vi "DB_LeeTHD_Graficas.vi"(8 "error in (no error)":errorcluster, 11 "ID_EQUIPO":i32=1) -> (0 "error out":errorcluster, 3 "THD out":T1)   [LabVIEW 2018]
uses:
  Controls/THD_cluster.ctl
  <vilib>/addons/database/Connection.llb/DB Tools Open Connec (Path).vi
  <vilib>/addons/database/Connection.llb/Conn Execute.vi
  <vilib>/addons/database/Recordset.llb/Rec Fetch Recordset Data (R).vi
  <vilib>/addons/database/Recordset.llb/Rec Destroy - Connection.vi
  <vilib>/addons/database/_DB Variant To Data/Database Variant To Data.xnode
  <vilib>/addons/database/NI_Database_API.lvlib
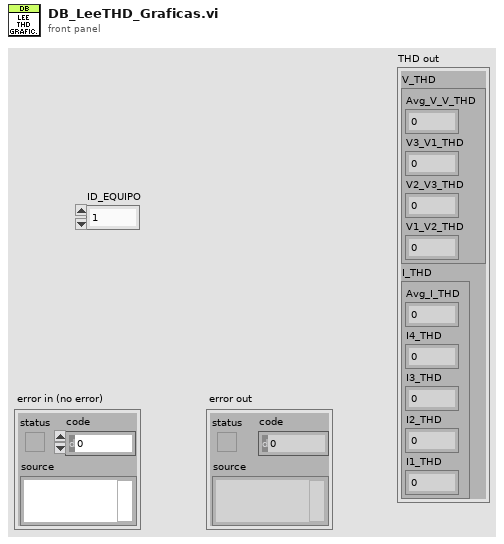
[diagram p1: front panel]
types:
  T1 = typedef "THD_cluster.ctl" = cluster{"V_THD":cluster{"Avg_V_V_THD":sgl, "V3_V1_THD":sgl, "V2_V3_THD":sgl, "V1_V2_THD":sgl}, "I_THD":cluster{"Avg_I_THD":sgl, "I4_THD":sgl, "I3_THD":sgl, "I2_THD":sgl, "I1_THD":sgl}}
  T2 = cluster{"Avg_I_THD":sgl, "I4_THD":sgl, "I3_THD":sgl, "I2_THD":sgl, "I1_THD":sgl}
  T3 = cluster{"Avg_V_V_THD":sgl, "V3_V1_THD":sgl, "V2_V3_THD":sgl, "V1_V2_THD":sgl}
  T4 = typedef "NI_Database_API.lvlib/Conn ObjectReference.ctl" = refnum<k1>
  T5 = typedef "NI_Database_API.lvlib/Rec ObjectReference.ctl" = refnum<k1>
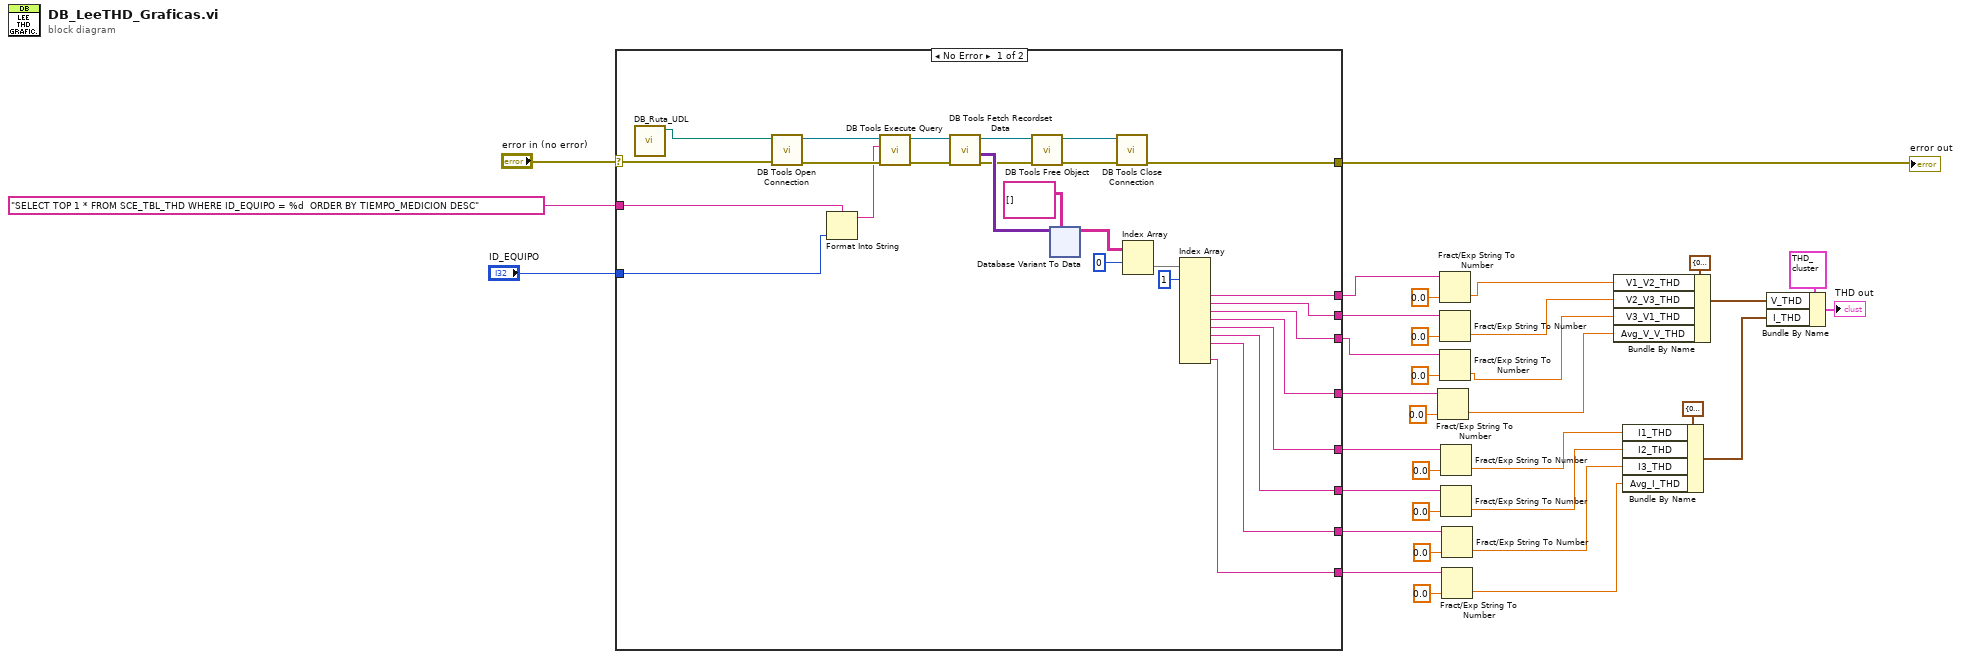
[diagram p0: block diagram]
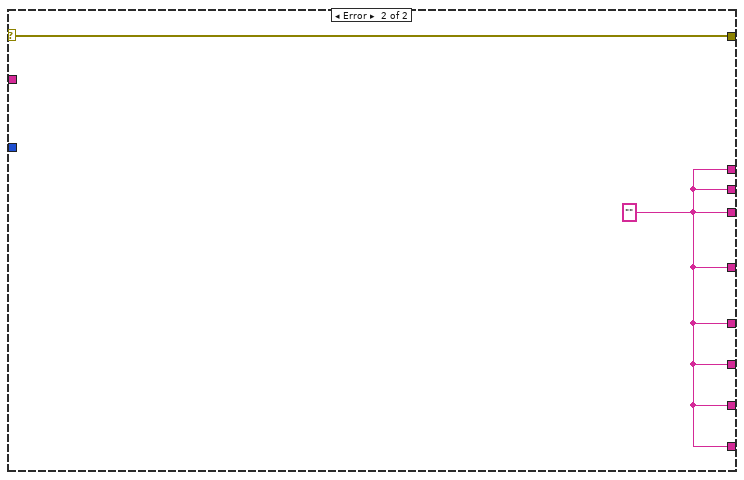
[diagram p2: hidden frame]
diagram:
  n1 = case shown="No Error" "error in (no error)" {
    selector: "error in (no error)" -> [w57 w108]
    tunnel: [w59 w108] -> w32
    tunnel: "SELECT TOP 1 * FROM SCE_TBL_THD WHERE ID_EQUIPO = %d  ORDER BY TIEMPO_MEDICION DESC" ("SQL") -> [w49 _]
    tunnel: [w45 w107] -> w30
    tunnel: [w44 w107] -> w26
    tunnel: [w43 w107] -> w25
    tunnel: "ID_EQUIPO" -> [w46 _]
    tunnel: [w41 w107] -> w21
    tunnel: [w42 w107] -> w20
    tunnel: [w40 w107] -> w19
    tunnel: [w38 w107] -> w9
    tunnel: [w37 w107] -> w7
    frame No Error {
      n2 = call "DB_Ruta_UDL.vi"() -> ("UDL ruta"=w36:path)  [unwired: 11 in]
      n3 = call-poly <vilib>:"DB Tools Open Connection.vi"("error in (no error)"=w57, "connection information"=w36) -> ("error out"=w62:errorcluster, "connection reference"=w60:T4)  [unwired: 6 in]
      n4 = Format Into String(format string=w49, w46) -> (resulting string=w48:string)  [unwired: 2 in, 1 out]
      n5 = call-poly <vilib>:"DB Tools Execute Query.vi"("error in (no error)"=w62, "SQL query"=w48, "connection reference"=w60) -> ("error out"=w58:errorcluster, "recordset reference"=w56:T5)  [unwired: 5 in]
      n6 = call-poly <vilib>:"DB Tools Fetch Recordset Data.vi"("error in (no error)"=w58, "recordset reference"=w56) -> ("error out"=w52:errorcluster, "recordset data"=w53:variant[][], "recordset reference out"=w55:T5)  [unwired: 3 in]
      n7 = call-poly <vilib>:"DB Tools Free Object.vi"("error in (no error)"=w52, "recordset reference"=w55) -> ("error out"=w61:errorcluster, "connection reference"=w35:T4)  [unwired: 8 in]
      n8 = xnode "Database Variant To Data"("database variant"=w53, "type"=string[][] []) -> ("data"=w51:string[][])  [unwired: 1 in, 1 out]
      n9 = call <vilib>:"DB Tools Close Connection.vi"("error in (no error)"=w61, "connection reference"=w35) -> ("error out"=w59:errorcluster)  [unwired: 5 in]
      n10 = Index Array(array=w51, index (row)=0 ("disabled index (col)")) -> (element=w47:string[])  [unwired: 1 in]
      n11 = Index Array(array=w47, index #1=1 ("index")) -> (element #3=w45:string, element #4=w44:string, element #5=w43:string, element #6=w38:string, element #7=w41:string, element #8=w42:string, element #9=w40:string, element #11=w37:string)  [unwired: 10 in, 3 out]
    }
    frame Error {
      w107 = ""
    }
  }
  "error out" <- w32
  n12 = Fract/Exp String To Number(string=w9, default (0 dbl)=sgl 0.0) -> (number=w5:sgl)  [unwired: 2 in, 1 out]
  n13 = Fract/Exp String To Number(string=w30, default (0 dbl)=sgl 0.0) -> (number=w17:sgl)  [unwired: 2 in, 1 out]
  n14 = Fract/Exp String To Number(string=w26, default (0 dbl)=sgl 0.0) -> (number=w16:sgl)  [unwired: 2 in, 1 out]
  n15 = Fract/Exp String To Number(string=w25, default (0 dbl)=sgl 0.0) -> (number=w15:sgl)  [unwired: 2 in, 1 out]
  n16 = Fract/Exp String To Number(string=w21, default (0 dbl)=sgl 0.0) -> (number=w14:sgl)  [unwired: 2 in, 1 out]
  n17 = Fract/Exp String To Number(string=w20, default (0 dbl)=sgl 0.0) -> (number=w13:sgl)  [unwired: 2 in, 1 out]
  n18 = Fract/Exp String To Number(string=w19, default (0 dbl)=sgl 0.0) -> (number=w12:sgl)  [unwired: 2 in, 1 out]
  n19 = Fract/Exp String To Number(string=w7, default (0 dbl)=sgl 0.0) -> (number=w6:sgl)  [unwired: 2 in, 1 out]
  n20 = Bundle By Name(cluster=T3 {"Avg_V_V_THD"=0.0, "V3_V1_THD"=0.0, "V2_V3_THD"=0.0, "V1_V2_THD"=0.0} ("V_THD"), "V1_V2_THD"=w17, "V2_V3_THD"=w16, "V3_V1_THD"=w15, "Avg_V_V_THD"=w5) -> (w18:T3)
  n21 = Bundle By Name(cluster=T2 {"Avg_I_THD"=0.0, "I4_THD"=0.0, "I3_THD"=0.0, "I2_THD"=0.0, "I1_THD"=0.0} ("I_THD"), "I1_THD"=w14, "I2_THD"=w13, "I3_THD"=w12, "Avg_I_THD"=w6) -> (w11:T2)
  n22 = Bundle By Name(cluster=T1 {"V_THD"={"Avg_V_V_THD"=0.0, "V3_V1_THD"=0.0, "V2_V3_THD"=0.0, "V1_V2_THD"=0.0}, "I_THD"={"Avg_I_THD"=0.0, "I4_THD"=0.0, "I3_THD"=0.0, "I2_THD"=0.0, "I1_THD"=0.0}} ("THD_cluster"), "V_THD"=w18, "I_THD"=w11) -> (→"THD out":T1)
